vi "FGV.vi"() -> ()   [LabVIEW 2019]
panel:
  out "Value out":string
  in  "Value In":string
  in  "Function":enum16{"Set Value", "Get Value"}(ring)
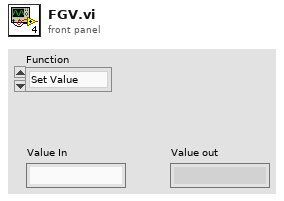
[diagram p1: front panel]
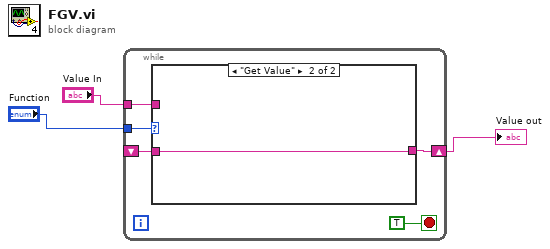
[diagram p0: block diagram]
diagram:
  n1 = while {
    shift-right: [w5] -> w1
    shift-left: _ -> [w4]
    tunnel: "Function" -> [w7]
    tunnel: "Value In" -> [w6]
    stop <- TRUE stop-if-true
    n2 = case shown="\"Get Value\"" w7 {
      tunnel: w6 -> [w9 _]
      tunnel: [w9 w10] -> w5
      tunnel: w4 -> [_ w10]
      frame "Set Value", Default {
      }
      frame "Get Value" {
      }
    }
  }
  "Value out" <- w1
